vi "Cellular_Uptake_Valve_Control.vi"() -> ()   [LabVIEW 2014]
uses:
  <vilib>/DAQmx/write.llb/DAQmx Write (Digital Bool 1Line 1Point).vi
panel:
  out "Trash":bool
  out "Medium":bool
  in  "Trash":bool
  in  "Dye":bool
  in  "LED":bool
  in  "Medium":bool
  in  "QUAKE VALVE":bool
  in  "Flush Medium":bool
  in  "Flush Dye":bool
  out "State":T1(ring)
  in  "LED  time:":dbl
  out "LED":bool
  out "Dye":bool
  out "QUAKE VALVE":bool
  in  "Before switch wait time:":dbl
  in  "Flow time":dbl
  in  "stop":bool
  # "Manual Control"
  # "Automatic Switch - set parameters:"
  # "ms"
  # "s"
  # "ms"
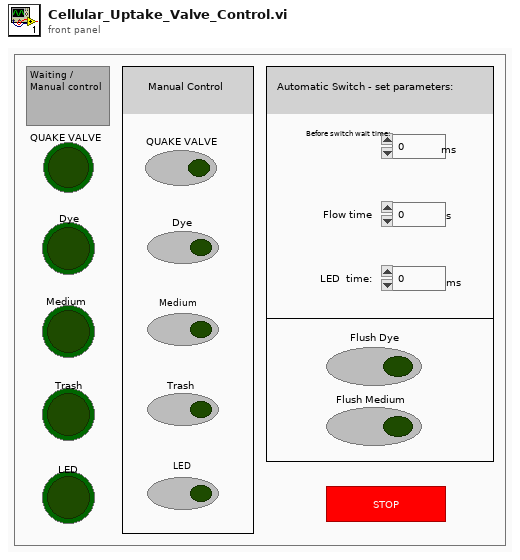
[diagram p1: front panel]
types:
  T1 = enum16{"Waiting / Manual control", "Flush Dye", "Flush Medium"}
  T2 = cluster{"1":bool, "2":bool, "Stop":bool, "LED":bool, "4":bool, "3":bool}
  T3 = cluster{"QUAKE VALVE":bool, "Dye":bool, "Medium":bool, "Trash":bool, "LED":bool, "stop":bool}
  T4 = cluster{"1":bool, "2":bool, "3":bool, "4":bool, "LED":bool, "stop":bool}
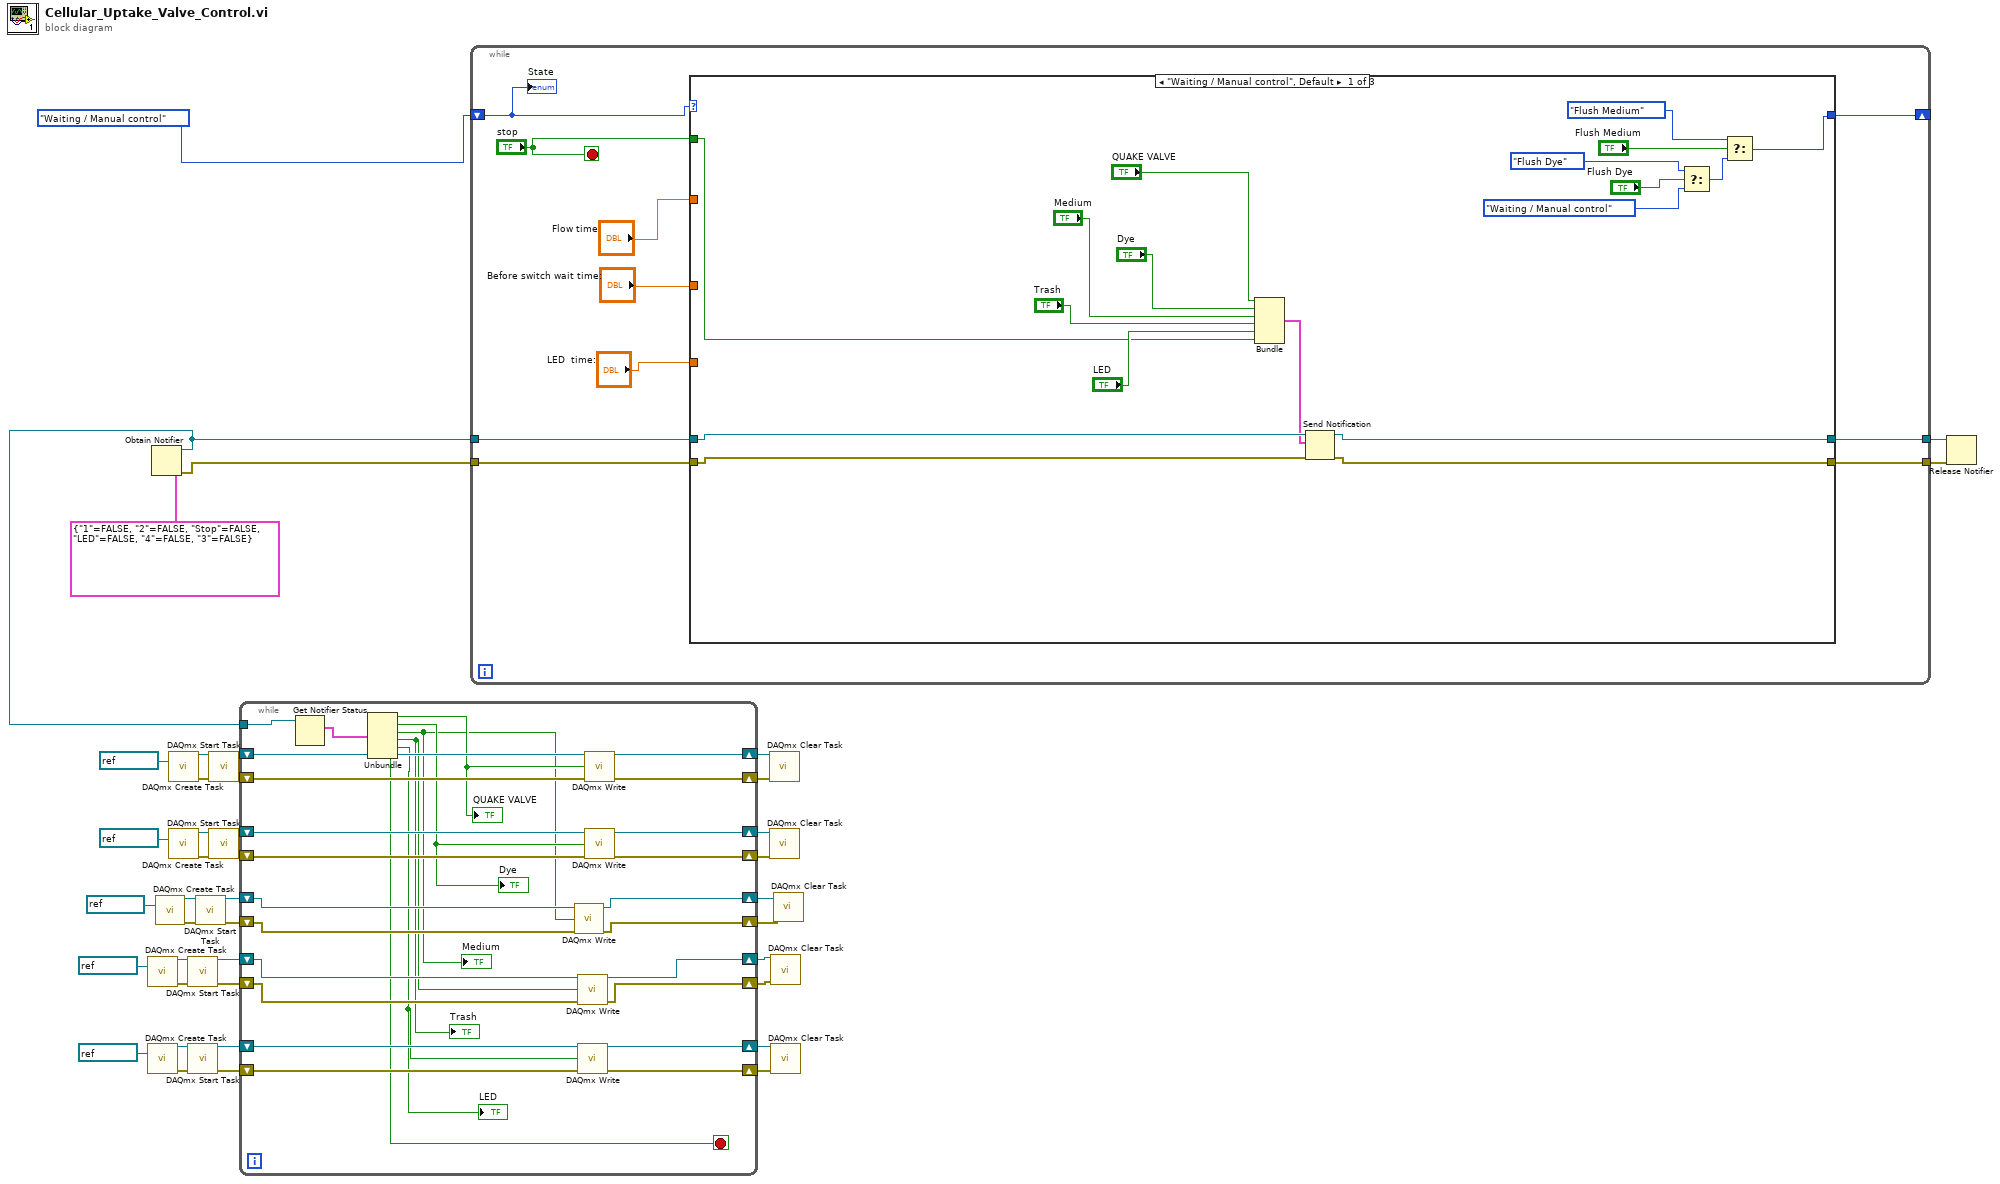
[diagram p0: block diagram]
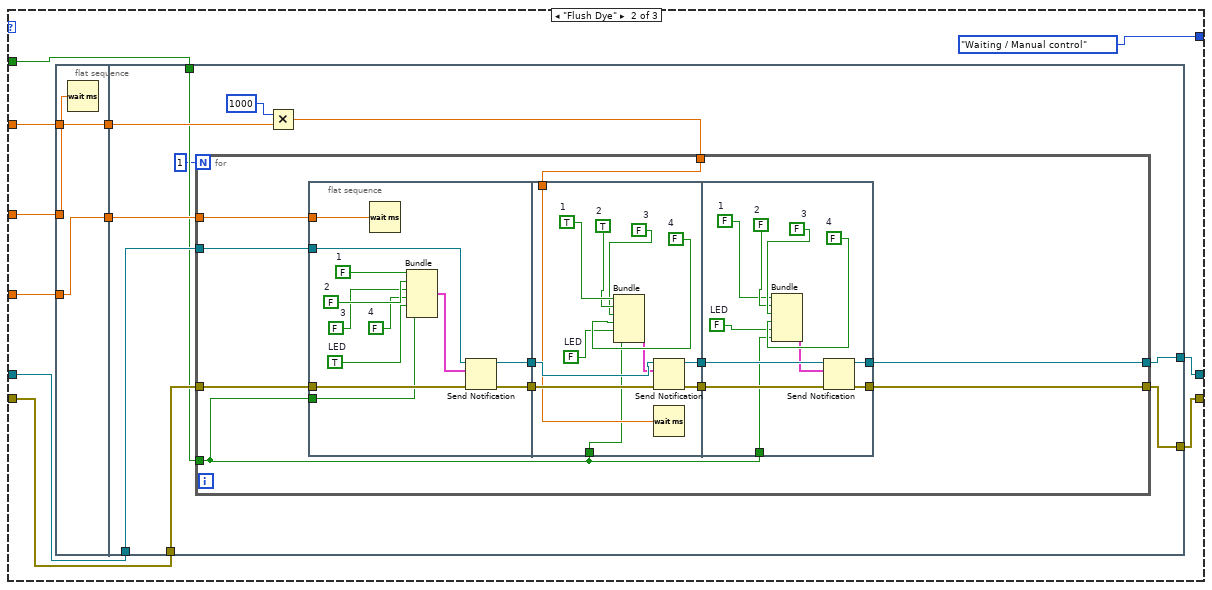
[diagram p2: hidden frame]
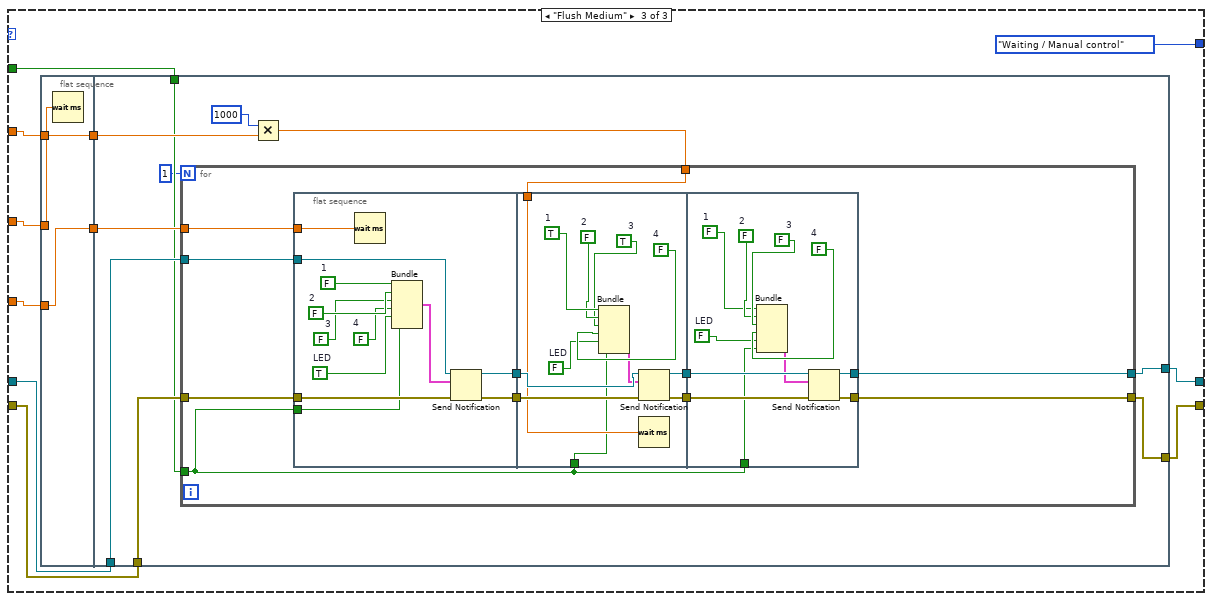
[diagram p3: hidden frame]
diagram:
  n1 = call <vilib>:"DAQmx Create Task.vi"("task to copy"=refnum<k21> "valve2") -> ("task out"=w18:refnum<k21>, "error out"=w17:errorcluster)  [unwired: 13 in]
  n2 = call <vilib>:"DAQmx Create Task.vi"("task to copy"=refnum<k21> "valve2") -> ("task out"=w15:refnum<k21>, "error out"=w14:errorcluster)  [unwired: 13 in]
  n3 = Obtain Notifier(notification data type=T2 {"1"=FALSE, "2"=FALSE, "Stop"=FALSE, "LED"=FALSE, "4"=FALSE, "3"=FALSE}) -> (notifier out=w22:refnum<notifier>, error out=w25:errorcluster)  [unwired: 3 in, 1 out]
  n4 = call <vilib>:"DAQmx Create Task.vi"("task to copy"=refnum<k21> "valve2") -> ("task out"=w21:refnum<k21>, "error out"=w20:errorcluster)  [unwired: 13 in]
  n5 = call <vilib>:"DAQmx Create Task.vi"("task to copy"=refnum<k21> "valve1") -> ("task out"=w35:refnum<k21>, "error out"=w36:errorcluster)  [unwired: 13 in]
  n6 = call <vilib>:"DAQmx Create Task.vi"("task to copy"=refnum<k21> "valve2") -> ("task out"=w40:refnum<k21>, "error out"=w39:errorcluster)  [unwired: 13 in]
  n7 = call <vilib>:"DAQmx Start Task.vi"("task/channels in"=w18, "error in"=w17) -> ("task out"=w10:refnum<k21>, "error out"=w9:errorcluster)  [unwired: 12 in]
  n8 = call <vilib>:"DAQmx Start Task.vi"("task/channels in"=w15, "error in"=w14) -> ("task out"=w8:refnum<k21>, "error out"=w7:errorcluster)  [unwired: 12 in]
  n9 = call <vilib>:"DAQmx Start Task.vi"("task/channels in"=w21, "error in"=w20) -> ("task out"=w12:refnum<k21>, "error out"=w11:errorcluster)  [unwired: 12 in]
  n10 = call <vilib>:"DAQmx Start Task.vi"("task/channels in"=w35, "error in"=w36) -> ("task out"=w34:refnum<k21>, "error out"=w33:errorcluster)  [unwired: 12 in]
  n11 = call <vilib>:"DAQmx Start Task.vi"("task/channels in"=w40, "error in"=w39) -> ("task out"=w32:refnum<k21>, "error out"=w31:errorcluster)  [unwired: 12 in]
  n12 = while {
    shift-right: [w63] -> w27
    shift-left: w31 -> [w66]
    shift-right: [w64] -> w28
    shift-left: w32 -> [w67]
    shift-right: [w62] -> w29
    shift-left: w33 -> [w68]
    shift-right: [w65] -> w30
    shift-left: w34 -> [w69]
    tunnel: w22 -> [w61]
    shift-right: [w52] -> w2
    shift-left: w12 -> [w60]
    shift-right: [w51] -> w1
    shift-left: w11 -> [w59]
    shift-right: [w54] -> w4
    shift-left: w10 -> [w58]
    shift-right: [w53] -> w3
    shift-left: w9 -> [w57]
    shift-right: [w50] -> w6
    shift-left: w8 -> [w56]
    shift-right: [w49] -> w5
    shift-left: w7 -> [w55]
    stop <- w47 stop-if-true
    n13 = Get Notifier Status(notifier=w61) -> (current notification=w48:T2)  [unwired: 1 in, 4 out]
    n14 = Unbundle(w48) -> ("1"=w45:bool, "2"=w44:bool, "Stop"=w43:bool, "LED"=w42:bool, "4"=w46:bool, "3"=w47:bool)
    "QUAKE VALVE" <- w45
    "Dye" <- w44
    "LED" <- w46
    "Medium" <- w43
    "Trash" <- w42
    n15 = call-poly <vilib>:"DAQmx Write.vi"("task/channels in"=w60, "data"=w43, "error in"=w59) -> ("task out"=w52:refnum<k21>, "error out"=w51:errorcluster)  [unwired: 10 in, 1 out]
    n16 = call-poly <vilib>:"DAQmx Write.vi"("task/channels in"=w58, "data"=w42, "error in"=w57) -> ("task out"=w54:refnum<k21>, "error out"=w53:errorcluster)  [unwired: 10 in, 1 out]
    n17 = call-poly <vilib>:"DAQmx Write.vi"("task/channels in"=w56, "data"=w46, "error in"=w55) -> ("task out"=w50:refnum<k21>, "error out"=w49:errorcluster)  [unwired: 10 in, 1 out]
    n18 = call-poly <vilib>:"DAQmx Write.vi"("task/channels in"=w69, "data"=w45, "error in"=w68) -> ("task out"=w65:refnum<k21>, "error out"=w62:errorcluster)  [unwired: 10 in, 1 out]
    n19 = call-poly <vilib>:"DAQmx Write.vi"("task/channels in"=w67, "data"=w44, "error in"=w66) -> ("task out"=w64:refnum<k21>, "error out"=w63:errorcluster)  [unwired: 10 in, 1 out]
  }
  n20 = while {
    shift-right: [w77] -> _
    shift-left: T1."Waiting / Manual control" ("State:") -> [w79]
    tunnel: w22 -> [w76]
    tunnel: w25 -> [w75]
    tunnel: [w74] -> w24
    tunnel: [w73] -> w23
    stop <- "stop" stop-if-true
    n21 = case shown="\"Waiting / Manual control\", Default" w79 {
      tunnel: "stop" -> [w80 w100 w175]
      tunnel: [w91 T1."Waiting / Manual control" ("State:") T1."Waiting / Manual control" ("State:")] -> w77
      tunnel: w76 -> [w90 w105 w171]
      tunnel: w75 -> [w88 w104 w170]
      tunnel: [w89 w99 w169] -> w74
      tunnel: [w87 w98 w168] -> w73
      tunnel: "Before switch wait time:" -> [_ w106 w173]
      tunnel: "Flow time" -> [_ w103 w174]
      tunnel: "LED  time:" -> [_ w102 w172]
      frame "Waiting / Manual control", Default {
        n22 = Bundle("QUAKE VALVE"="QUAKE VALVE", "Dye"="Dye", "Medium"="Medium", "Trash"="Trash", "LED"="LED", "stop"=w80) -> (w86:T3)  [unwired: 1 in]
        n23 = Send Notification(notification=w86, notifier=w90, error in (no error)=w88) -> (notifier out=w89:refnum<notifier>, error out=w87:errorcluster)
        n24 = Select(t=T1."Flush Dye" ("State:"), s="Flush Dye", f=T1."Waiting / Manual control" ("State:")) -> (s? t:f=w93:T1)
        n25 = Select(t=T1."Flush Medium" ("State:"), s="Flush Medium", f=w93) -> (s? t:f=w91:T1)
      }
      frame "Flush Dye" {
        n26 = flat-sequence {
          tunnel: [w110] -> w107
          tunnel: w106 -> [w111]
          tunnel: w103 -> [w110]
          tunnel: w102 -> [w109]
          tunnel: [w109] -> w101
          tunnel: w105 -> [w121]
          tunnel: w104 -> [w120]
          tunnel: [w119] -> w99
          tunnel: [w118] -> w98
          tunnel: w107 -> [w117]
          tunnel: w101 -> [w114]
          tunnel: w100 -> [w113]
          frame #0 {
            n27 = Wait (ms)(milliseconds to wait=w111) -> ()  [unwired: 1 out]
          }
          frame #1 {
            n28 = Multiply(x=1000, y=w117) -> (x*y=w115:dbl)
            n29 = for {
              N: 1 -> [_]
              tunnel: w121 -> [w128]
              tunnel: w120 -> [w127]
              tunnel: [w123] -> w118
              tunnel: [w124] -> w119
              tunnel: w113 -> [w125]
              tunnel: w114 -> [w126]
              tunnel: w115 -> [w122]
              n30 = flat-sequence {
                tunnel: [w143] -> w132
                tunnel: [w142] -> w131
                tunnel: w125 -> [w134]
                tunnel: w128 -> [w133]
                tunnel: w127 -> [w144]
                tunnel: w126 -> [w140]
                tunnel: [w153] -> w130
                tunnel: w132 -> [w154]
                tunnel: [w155] -> w129
                tunnel: w131 -> [w156]
                tunnel: w125 -> [w145]
                tunnel: w122 -> [w152]
                tunnel: w130 -> [w167]
                tunnel: w129 -> [w166]
                tunnel: w125 -> [w158]
                tunnel: [w165] -> w124
                tunnel: [w164] -> w123
                frame #0 {
                  w137 = FALSE  # 3
                  w136 = FALSE  # 4
                  w135 = TRUE  # LED
                  w138 = FALSE  # 2
                  w139 = FALSE  # 1
                  n31 = Wait (ms)(milliseconds to wait=w140) -> ()  [unwired: 1 out]
                  n32 = Bundle("1"=w139, "2"=w138, "3"=w137, "4"=w136, "LED"=w135, "stop"=w134) -> (w141:T4)  [unwired: 1 in]
                  n33 = Send Notification(notification=w141, notifier=w133, error in (no error)=w144) -> (notifier out=w143:refnum<notifier>, error out=w142:errorcluster)
                }
                frame #1 {
                  w149 = FALSE  # 3
                  w148 = FALSE  # 4
                  w147 = FALSE  # LED
                  w150 = TRUE  # 2
                  w151 = TRUE  # 1
                  n34 = Bundle("1"=w151, "2"=w150, "3"=w149, "4"=w148, "LED"=w147, "stop"=w145) -> (w146:T4)  [unwired: 1 in]
                  n35 = Send Notification(notification=w146, notifier=w154, error in (no error)=w156) -> (notifier out=w153:refnum<notifier>, error out=w155:errorcluster)
                  n36 = Wait (ms)(milliseconds to wait=w152) -> ()  [unwired: 1 out]
                }
                frame #2 {
                  w163 = FALSE  # 3
                  w160 = FALSE  # 4
                  w159 = FALSE  # LED
                  w162 = FALSE  # 2
                  w161 = FALSE  # 1
                  n37 = Bundle("1"=w161, "2"=w162, "3"=w163, "4"=w160, "LED"=w159, "stop"=w158) -> (w157:T4)  [unwired: 1 in]
                  n38 = Send Notification(notification=w157, notifier=w167, error in (no error)=w166) -> (notifier out=w165:refnum<notifier>, error out=w164:errorcluster)
                }
              }
            }
          }
        }
      }
      frame "Flush Medium" {
        n39 = flat-sequence {
          tunnel: [w180] -> w177
          tunnel: w173 -> [w181]
          tunnel: w174 -> [w180]
          tunnel: w172 -> [w179]
          tunnel: [w179] -> w176
          tunnel: w171 -> [w191]
          tunnel: w170 -> [w190]
          tunnel: [w189] -> w169
          tunnel: [w188] -> w168
          tunnel: w177 -> [w187]
          tunnel: w176 -> [w184]
          tunnel: w175 -> [w183]
          frame #0 {
            n40 = Wait (ms)(milliseconds to wait=w181) -> ()  [unwired: 1 out]
          }
          frame #1 {
            n41 = Multiply(x=1000, y=w187) -> (x*y=w185:dbl)
            n42 = for {
              N: 1 -> [_]
              tunnel: w191 -> [w198]
              tunnel: w190 -> [w197]
              tunnel: [w193] -> w188
              tunnel: [w194] -> w189
              tunnel: w183 -> [w195]
              tunnel: w184 -> [w196]
              tunnel: w185 -> [w192]
              n43 = flat-sequence {
                tunnel: [w213] -> w202
                tunnel: [w212] -> w201
                tunnel: w195 -> [w204]
                tunnel: w198 -> [w203]
                tunnel: w197 -> [w214]
                tunnel: w196 -> [w210]
                tunnel: [w223] -> w200
                tunnel: w202 -> [w224]
                tunnel: [w225] -> w199
                tunnel: w201 -> [w226]
                tunnel: w195 -> [w215]
                tunnel: w192 -> [w222]
                tunnel: w200 -> [w237]
                tunnel: w199 -> [w236]
                tunnel: w195 -> [w228]
                tunnel: [w235] -> w194
                tunnel: [w234] -> w193
                frame #0 {
                  w207 = FALSE  # 3
                  w206 = FALSE  # 4
                  w205 = TRUE  # LED
                  w208 = FALSE  # 2
                  w209 = FALSE  # 1
                  n44 = Wait (ms)(milliseconds to wait=w210) -> ()  [unwired: 1 out]
                  n45 = Bundle("1"=w209, "2"=w208, "3"=w207, "4"=w206, "LED"=w205, "stop"=w204) -> (w211:T4)  [unwired: 1 in]
                  n46 = Send Notification(notification=w211, notifier=w203, error in (no error)=w214) -> (notifier out=w213:refnum<notifier>, error out=w212:errorcluster)
                }
                frame #1 {
                  w219 = TRUE  # 3
                  w218 = FALSE  # 4
                  w217 = FALSE  # LED
                  w220 = FALSE  # 2
                  w221 = TRUE  # 1
                  n47 = Bundle("1"=w221, "2"=w220, "3"=w219, "4"=w218, "LED"=w217, "stop"=w215) -> (w216:T4)  [unwired: 1 in]
                  n48 = Send Notification(notification=w216, notifier=w224, error in (no error)=w226) -> (notifier out=w223:refnum<notifier>, error out=w225:errorcluster)
                  n49 = Wait (ms)(milliseconds to wait=w222) -> ()  [unwired: 1 out]
                }
                frame #2 {
                  w233 = FALSE  # 3
                  w230 = FALSE  # 4
                  w229 = FALSE  # LED
                  w232 = FALSE  # 2
                  w231 = FALSE  # 1
                  n50 = Bundle("1"=w231, "2"=w232, "3"=w233, "4"=w230, "LED"=w229, "stop"=w228) -> (w227:T4)  [unwired: 1 in]
                  n51 = Send Notification(notification=w227, notifier=w237, error in (no error)=w236) -> (notifier out=w235:refnum<notifier>, error out=w234:errorcluster)
                }
              }
            }
          }
        }
      }
    }
    "State" <- w79
  }
  n52 = call <vilib>:"DAQmx Clear Task.vi"("task in"=w30, "error in"=w29) -> ()  [unwired: 13 in, 1 out]
  n53 = call <vilib>:"DAQmx Clear Task.vi"("task in"=w28, "error in"=w27) -> ()  [unwired: 13 in, 1 out]
  n54 = call <vilib>:"DAQmx Clear Task.vi"("task in"=w4, "error in"=w3) -> ()  [unwired: 13 in, 1 out]
  n55 = call <vilib>:"DAQmx Clear Task.vi"("task in"=w6, "error in"=w5) -> ()  [unwired: 13 in, 1 out]
  n56 = call <vilib>:"DAQmx Clear Task.vi"("task in"=w2, "error in"=w1) -> ()  [unwired: 13 in, 1 out]
  n57 = Release Notifier(notifier=w24, error in (no error)=w23) -> ()  [unwired: 1 in, 3 out]
